vi "shock.vi"() -> ()   [LabVIEW 2018]
uses:
  <vilib>/DAQmx/write.llb/DAQmx Write (Analog Wfm 1Chan NSamp).vi
  <vilib>/DAQmx/miscellaneous.llb/DAQmx Fill In Error Info.vi
  <vilib>/DAQmx/create/channels.llb/DAQmx Create Channel (AO-Voltage-Basic).vi
  <vilib>/DAQmx/configure/timing.llb/DAQmx Timing (Sample Clock).vi
  <vilib>/measure/NI_MABase.lvlib
  <resource>/objmgr/daqmx.rc
panel:
  in  "Tab Control":enum32{"Settings", "Advanced"}(tab)
  in  "frequency":dbl=0.5 format="%0.2p"
  in  "Voltage [V]":dbl=5.0 format="%0.2p"
  in  "duty cycle (%)":dbl=20.0 format="%0.2f"
  in  "duration [s]":u32
  in  "phase":dbl format="%.2p"
  out "State 2":enum16{"shock", "end", "listen", "init"}(ring)=enum."end"
  in  "signal type":T1(ring)=enum."Square Wave"
  out "Output Signal":waveform(dbl)(graph)={"t0"=timestamp(52855.0 s since 1904-01-01), "dt"=0.001, "Y"=array[1000 elements]}
  in  "Shock":bool
  in  "stop":bool
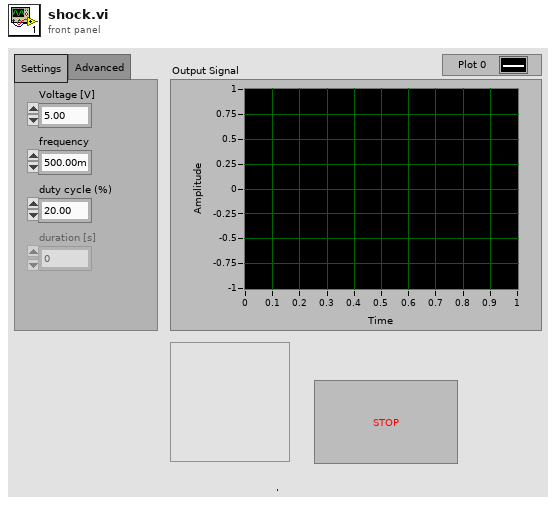
[diagram p1: front panel]
types:
  T1 = enum16{"Sine Wave", "Triangle Wave", "Square Wave", "Sawtooth Wave"}
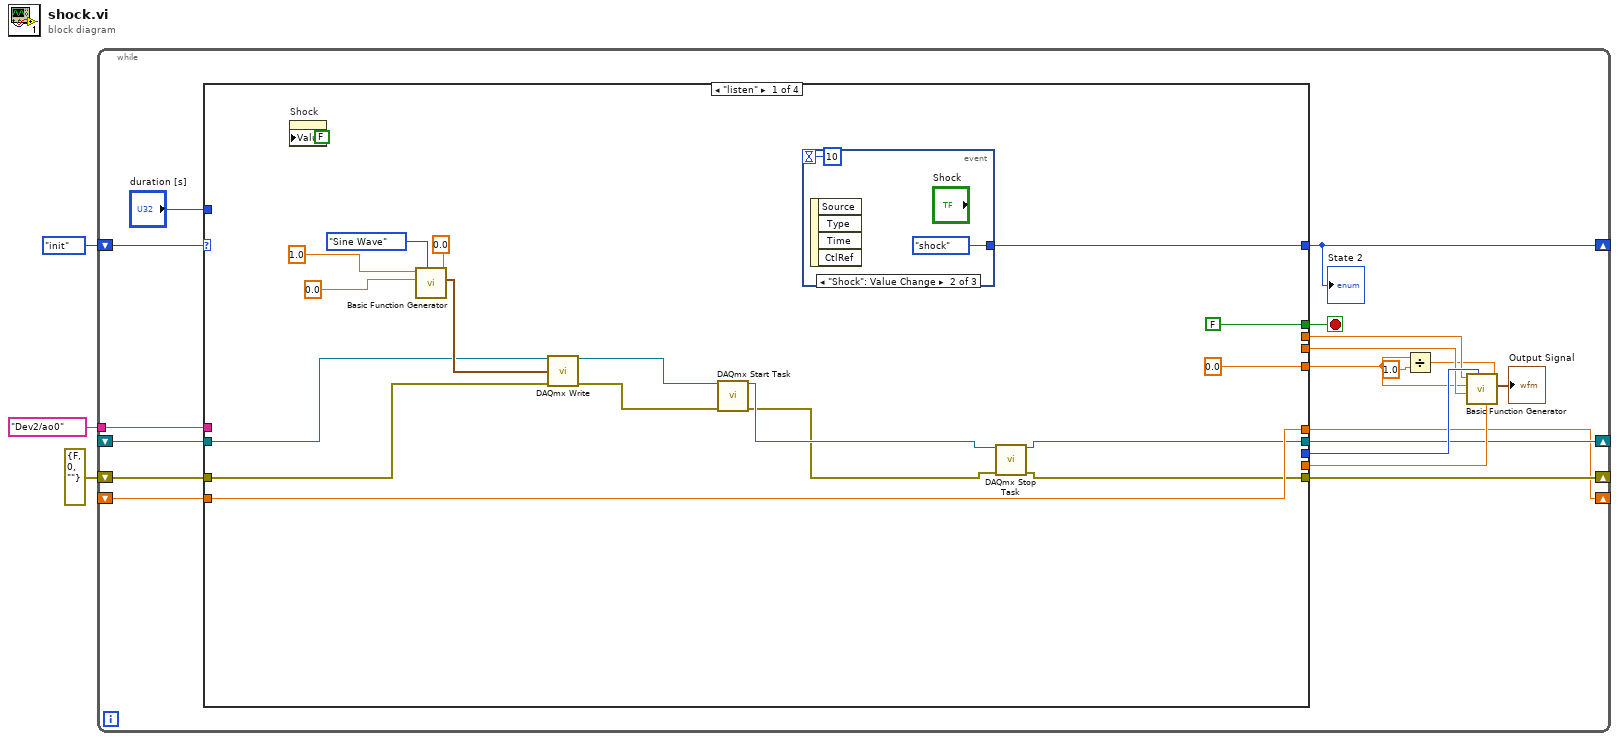
[diagram p0: block diagram]
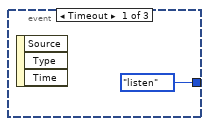
[diagram p2: hidden frame]
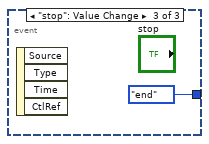
[diagram p3: hidden frame]
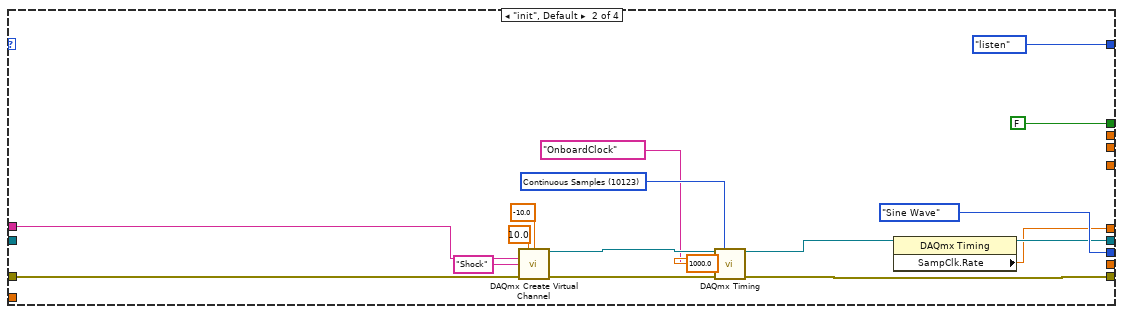
[diagram p4: hidden frame]
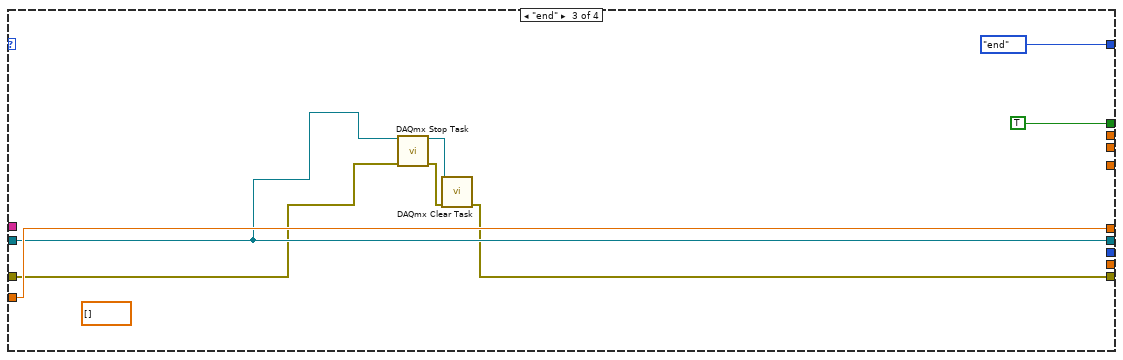
[diagram p5: hidden frame]
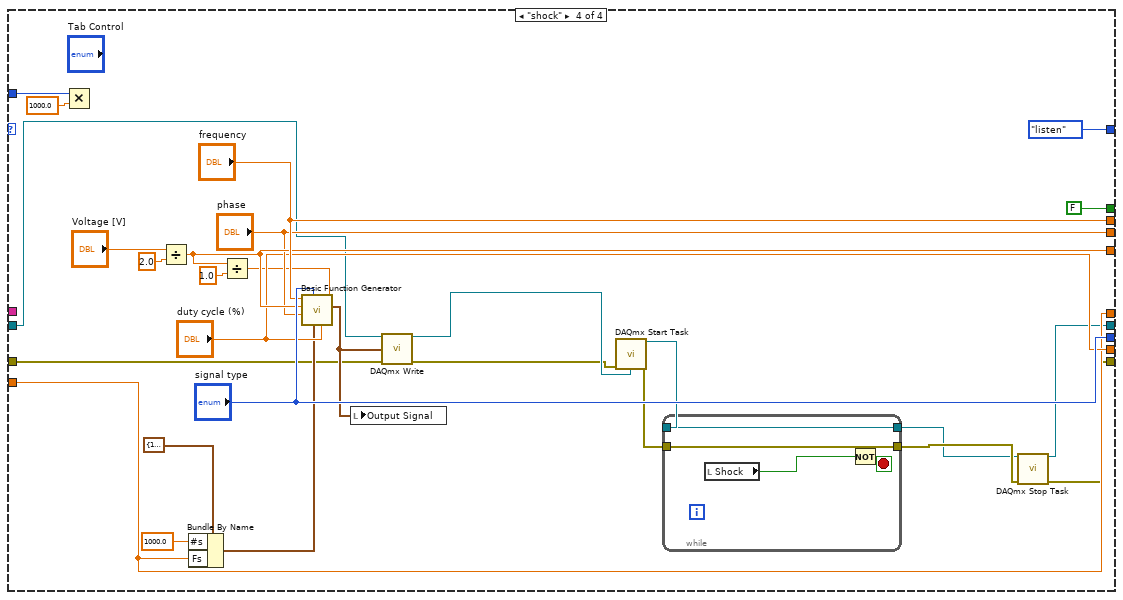
[diagram p6: hidden frame]
diagram:
  n1 = while {
    shift-right: [w20] -> _
    shift-left: enum16{"shock", "end", "listen", "init"}."init" ("State") -> [w21]
    shift-right: [w13] -> _
    shift-left: errorcluster {"status"=FALSE, "code"=0, "source"=""} ("error out") -> [w12]
    tunnel: tag "Dev2/ao0" ("physical channels") -> [w8]
    shift-right: [w7] -> _
    shift-left: _ -> [w6]
    shift-right: [w5] -> _
    shift-left: _ -> [w4]
    stop <- w22 stop-if-true
    n2 = case shown="\"listen\"" w21 {
      tunnel: [FALSE FALSE TRUE FALSE] -> w22
      tunnel: [w40 enum16{"shock", "end", "listen", "init"}."listen" ("State 2") enum16{"shock", "end", "listen", "init"}."end" ("State 2") enum16{"shock", "end", "listen", "init"}."listen" ("State 2")] -> w20
      tunnel: [_ T1."Sine Wave" ("signal type") _ "signal type"] -> w19
      tunnel: [_ _ _ "frequency"] -> w18
      tunnel: [0.0 ("amplitude") _ _ w91] -> w10
      tunnel: [_ _ _ "phase"] -> w17
      tunnel: [_ _ _ "duty cycle (%)"] -> w16
      tunnel: "duration [s]" -> [_ _ _ w94]
      tunnel: [w25 w47 w66 w71] -> w7
      tunnel: [w23 w54 w62 w70] -> w13
      tunnel: w12 -> [w27 w58 w63 w78]
      tunnel: w8 -> [_ w57 _ _]
      tunnel: w6 -> [w28 _ w66 w79]
      tunnel: [w36 w46 w67 w88] -> w5
      tunnel: w4 -> [w36 _ w67 w88]
      frame "listen" {
        n3 = property on="Shock" class="Bool (strict)"("Value"=FALSE ("Shock")) -> ()  [unwired: 2 in, 2 out]
        n4 = call <vilib>:"Basic Function Generator.vi"("offset"=0.0, "signal type"=T1."Sine Wave", "amplitude"=0.0, "frequency"=1.0) -> ("signal out"=w35:waveform(dbl))  [unwired: 5 in, 2 out]
        n5 = call-poly <vilib>:"DAQmx Write.vi"("task/channels in"=w28, "data"=w35, "error in"=w27) -> ("task out"=w30:refnum<k21>, "error out"=w29:errorcluster)  [unwired: 10 in, 1 out]
        n6 = call <vilib>:"DAQmx Start Task.vi"("task/channels in"=w30, "error in"=w29) -> ("task out"=w26:refnum<k21>, "error out"=w24:errorcluster)  [unwired: 12 in]
        n7 = event shown="[1] \"Shock\": Value Change" {
          selector: _ -> [_ _ _]
          dyn-events: _ -> [_ _ _]
          timeout: 10 -> [_ _ _]
          tunnel: [enum16{"shock", "end", "listen", "init"}."listen" ("State 2") enum16{"shock", "end", "listen", "init"}."shock" ("State 2") enum16{"shock", "end", "listen", "init"}."end" ("State 2")] -> w40
          event Timeout {
            n8 = event-data() -> ()  [unwired: 1 in, 3 out]
          }
          event "Shock": Value Change {
            n9 = event-data() -> ()  [unwired: 1 in, 4 out]
          }
          event "stop": Value Change {
            n10 = event-data() -> ()  [unwired: 1 in, 4 out]
          }
        }
        n11 = call <vilib>:"DAQmx Stop Task.vi"("task/channels in"=w26, "error in"=w24) -> ("task out"=w25:refnum<k21>, "error out"=w23:errorcluster)  [unwired: 12 in]
      }
      frame "init", Default {
        w53 = 10123 items=["Finite Samples"=10178, "Continuous Samples"=10123, "Hardware Timed Single Point"=12522] ("sample mode")
        n12 = call-poly <vilib>:"DAQmx Create Virtual Channel.vi"("maximum value"=10.0, "minimum value"=-10.0, "physical channels"=w57, "name to assign"="Shock", "error in"=w58) -> ("task out"=w56:refnum<k21>, "error out"=w55:errorcluster)  [unwired: 9 in]
        n13 = call-poly <vilib>:"DAQmx Timing.vi"("task/channels in"=w56, "sample mode"=w53, "rate"=1000.0, "source"=tag "OnboardClock", "error in"=w55) -> ("task out"=w48:refnum<k21>, "error out"=w54:errorcluster)  [unwired: 9 in]
        n14 = property class="DAQmx Timing"(reference=w48) -> (reference out=w47:refnum<k21>, "SampClk.Rate"=w46:dbl)  [unwired: 1 in, 1 out]
      }
      frame "end" {
        (unwired) dbl[] [] ("Y")
        n15 = call <vilib>:"DAQmx Stop Task.vi"("task/channels in"=w66, "error in"=w63) -> ("task out"=w64:refnum<k21>, "error out"=w65:errorcluster)  [unwired: 12 in]
        n16 = call <vilib>:"DAQmx Clear Task.vi"("task in"=w64, "error in"=w65) -> ("error out"=w62:errorcluster)  [unwired: 13 in]
      }
      frame "shock" {
        n17 = Multiply(x=w94, y=1000.0) -> ()  [unwired: 1 out]
        n18 = Divide(x="Voltage [V]", y=2.0) -> (x/y=w91:dbl)
        n19 = Bundle By Name(cluster=cluster{"Fs":dbl, "#s":dbl} {"Fs"=1000.0, "#s"=1000.0} ("sampling info"), "#s"=1000.0, "Fs"=w88) -> (w85:cluster{"Fs":dbl, "#s":dbl})
        n20 = Divide(x=w91, y=1.0 ("x")) -> (x/y=w81:dbl)
        n21 = call <vilib>:"Basic Function Generator.vi"("offset"=w81, "square wave duty cycle (%)"="duty cycle (%)", "sampling info"=w85, "signal type"="signal type", "phase"="phase", "amplitude"=w91, "frequency"="frequency") -> ("signal out"=w84:waveform(dbl))  [unwired: 2 in, 2 out]
        n22 = local write "Output Signal"(w84) -> ()
        n23 = call-poly <vilib>:"DAQmx Write.vi"("task/channels in"=w79, "data"=w84, "error in"=w78) -> ("task out"=w77:refnum<k21>, "error out"=w76:errorcluster)  [unwired: 10 in, 1 out]
        n24 = call <vilib>:"DAQmx Start Task.vi"("task/channels in"=w77, "error in"=w76) -> ("task out"=w75:refnum<k21>, "error out"=w74:errorcluster)  [unwired: 12 in]
        n25 = while {
          tunnel: w75 -> [w101]
          tunnel: [w101] -> w72
          tunnel: w74 -> [w100]
          tunnel: [w100] -> w73
          stop <- w98 stop-if-true
          n26 = local read "Shock"() -> (w99:bool)
          n27 = Not(x=w99) -> (.not. x?=w98:bool)
        }
        n28 = call <vilib>:"DAQmx Stop Task.vi"("task/channels in"=w72, "error in"=w73) -> ("task out"=w71:refnum<k21>, "error out"=w70:errorcluster)  [unwired: 12 in]
      }
    }
    "State 2" <- w20
    n29 = Divide(x=w10, y=1.0) -> (x/y=w11:dbl)
    n30 = call <vilib>:"Basic Function Generator.vi"("offset"=w11, "square wave duty cycle (%)"=w16, "signal type"=w19, "phase"=w17, "amplitude"=w10, "frequency"=w18) -> ("signal out"=→"Output Signal":waveform(dbl))  [unwired: 3 in, 2 out]
  }
